vi "Load Instrument Classes.vi"(8 "error in (no error)":errorcluster, 11 "C.E.":refnum<class "Control Experiment.lvclass">) -> (0 "error out":errorcluster, 1 "unresolved":string[](array[string]), 2 "cancelled":bool, 3 "Control Experiment":refnum<class "Control Experiment.lvclass">)   [LabVIEW 2019, in "Control Experiment.lvclass"]
uses:
  Control Experiment.lvclass
  Typedefs/Instrument Class Rings--Cluster.ctl
  <userlib>/LevyLab/Instrument Framework/Instrument/Instrument.lvclass
  C:/Program Files/National Instruments/LabVIEW 2019/vi.lib/JKI/JKI SMO/SMO/SMO.lvclass
  Control Experiment.lvclass/Control Experiment.ctl
  Typedefs/Instrument Classes--cluster.ctl
  <userlib>/LevyLab/Instrument Framework/Instrument Types/Lockin/Instrument.LockinAPI.lvclass
  <userlib>/LevyLab/Instrument Framework/Instrument Types/Amplifier/Instrument.Amplifier.lvclass
  <userlib>/LevyLab/Instrument Framework/Instrument Types/Cryostat/Instrument.Cryostat.lvclass
  <userlib>/LevyLab/Instrument Framework/Instrument Types/CBridge/Instrument.CBridge.lvclass
  <userlib>/LevyLab/Instrument Framework/Instrument Types/Delay Line/Instrument.DelayLine.lvclass
  <userlib>/LevyLab/Instrument Framework/Instrument Types/Strain/Instrument.Strain.lvclass
  <userlib>/LevyLab/Instrument Framework/Instrument Types/VNA/Instrument.VNA.lvclass
  <userlib>/LevyLab/Instrument Framework/Instrument Types/VSource/Instrument.VSource.lvclass
  Typedefs/Instrument Types--enum.ctl
  <userlib>/LevyLab/Instrument Framework/Instrument/Instrument.lvclass/Instrument.ctl
  <vilib>/Utility/Data Type/NI_Data Type.lvlib
  Attributes/Instrument Attributes.lvlib
  <vilib>/JKI/JKI SMO/URI Parsing/URI.lvlib
panel:
  in  "DAQ":refnum<visa-resource-name>
  in  "Instrument Addresses":T1 caption="Instruments"
  in  "OK":bool
  in  "Instrument Classes":T2 {"Amplifier" items=["", "Krohn-Hite-7008"]; "DAQ" items=["", "Lockin"]; "Strain Cell" items=["", "RP100"]; "Capacitance" items=["", "AH2500"]; "Level" items=["", "Cryostation", "OxfordVRM", "OptiCool", "PPMS", "PPMS1", "PPMS2", "PPMS3"]; "Rotator" items=["", "Cryostation", "OxfordVRM", "OptiCool", "PPMS", "PPMS1", "PPMS2", "PPMS3"]; "Magnet" items=["", "Cryostation", "OxfordVRM", "OptiCool", "PPMS", "PPMS1", "PPMS2", "PPMS3"]; "Temperature" items=["", "Cryostation", "OxfordVRM", "OptiCool", "PPMS", "PPMS1", "PPMS2", "PPMS3"]}
  out "Status":string
  # "1. Choose / Confirm Instrument Classes"
  # "2. Choose / Confirm Remote Instruments"
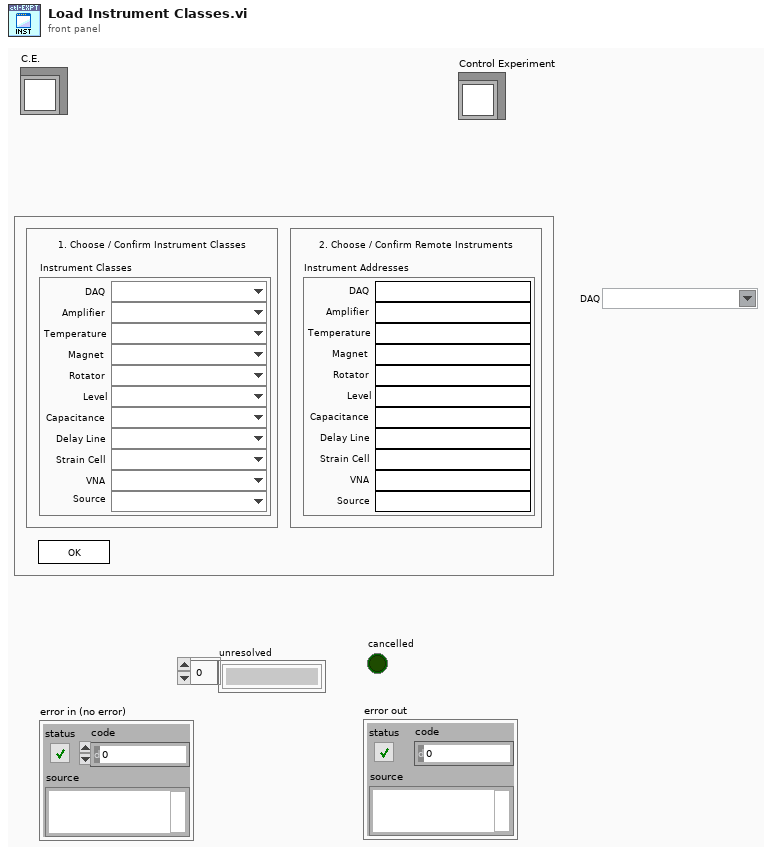
[diagram p1: front panel]
types:
  T1 = cluster{"DAQ":string, "Amplifier":string, "Temperature":string, "Magnet":string, "Rotator":string, "Level":string, "Capacitance Bridge":string, "Delay Line":string, "Strain Cell":string, "VNA":string, "Source":string}
  T2 = typedef "Control Experiment.lvclass/Instrument Class Rings--Cluster.ctl" = cluster{"DAQ":u16, "Amplifier":u16, "Temperature":u16, "Magnet":u16, "Rotator":u16, "Level":u16, "Capacitance":u16, "Delay Line":u16, "Strain Cell":u16, "VNA":u16, "Source":u16}
  T3 = enum32{"Invalid", "Standard", "Closed", "Hidden", "Minimized", "Maximized"}
  T4 = enum32{"invalid app kind", "Development System", "Run Time System", "Student Edition", "Embedded LabVIEW", "Evaluation", "Custom"}
  T5 = typedef "Control Experiment.lvclass/Instrument Classes--cluster.ctl" = cluster{"DAQ":refnum<class "Instrument.LockinAPI.lvclass">, "Amplifier":refnum<class "Instrument.Amplifier.lvclass">, "Temperature":refnum<class "Instrument.Cryostat.lvclass">, "Magnet":refnum<class "Instrument.Cryostat.lvclass">, "Rotator":refnum<class "Instrument.Cryostat.lvclass">, "Level":refnum<class "Instrument.Cryostat.lvclass">, "Capacitance":refnum<class "Instrument.CBridge.lvclass">, "Delay Line":refnum<class "Instrument.DelayLine.lvclass">, "Strain Cell":refnum<class "Instrument.Strain.lvclass">, "VNA":refnum<class "Instrument.VNA.lvclass">, "Source":refnum<class "Instrument.VSource.lvclass">}
  T6 = typedef "Control Experiment.lvclass/Instrument Types--enum.ctl" = enum16{"DAQ", "Amplifier", "Temperature", "Magnet", "Rotator", "Level", "Capacitance", "Delay Line", "Strain Cell", "VNA", "Source"}
  T7 = cluster{"Core":cluster{"Current VI Reference":refnum<vi>, "Close Panel on Exit?":bool}, "C.E.":refnum<class "Control Experiment.lvclass">, "Instruments":refnum<vi>, "Addresses":refnum<vi>, "Instrument Class Rings":refnum<vi>[], "Installed Instruments":refnum<class "Instrument.lvclass">[], "Cast Instruments":refnum<class "Instrument.lvclass">[]}
  T8 = cluster{"Current VI Reference":refnum<vi>, "Close Panel on Exit?":bool}
  T9 = enum32{"Bad", "Idle", "Run top level", "Running"}
  T10 = typedef "Control Experiment.lvclass/Instruments--cluster.ctl" = cluster{"class path":path, "Address":string, "Type":T6}
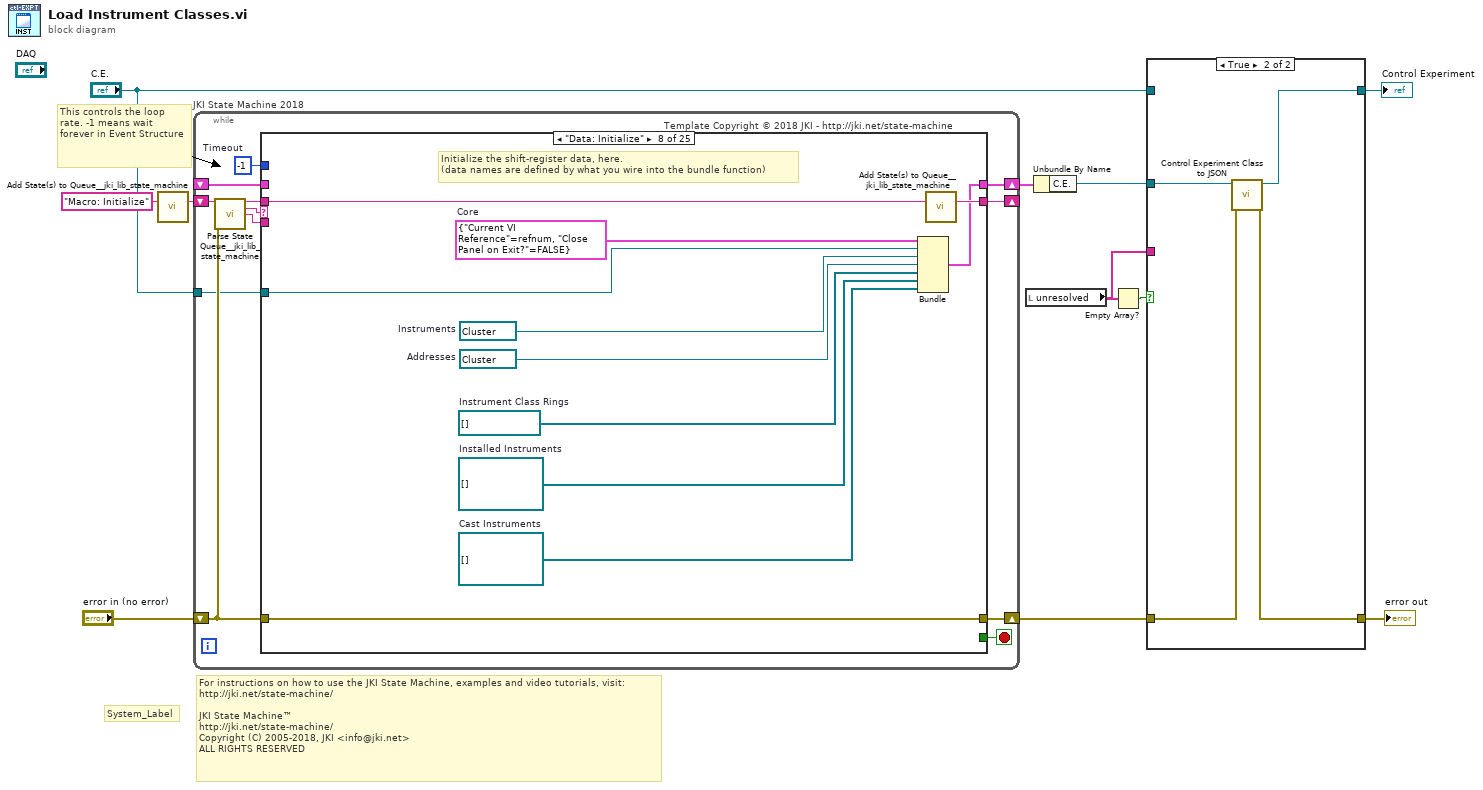
[diagram p0: block diagram]
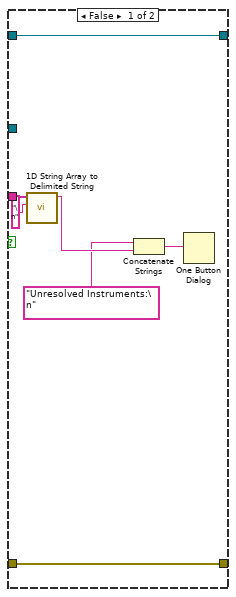
[diagram p2: hidden frame]
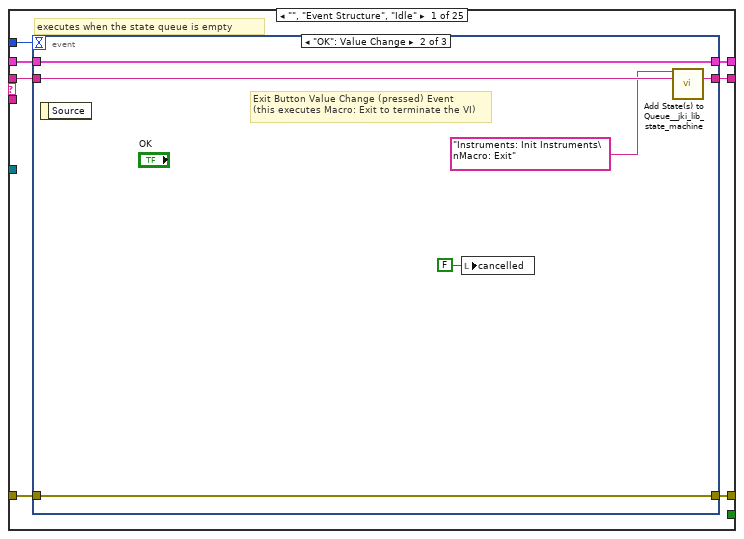
[diagram p3: hidden frame]
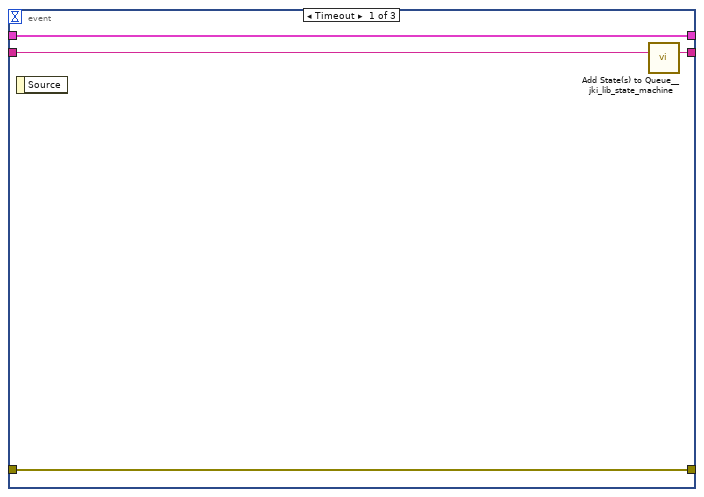
[diagram p4: hidden frame]
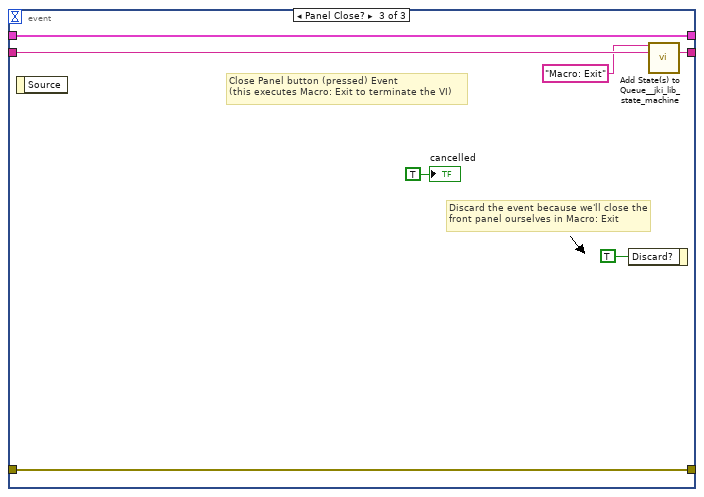
[diagram p5: hidden frame]
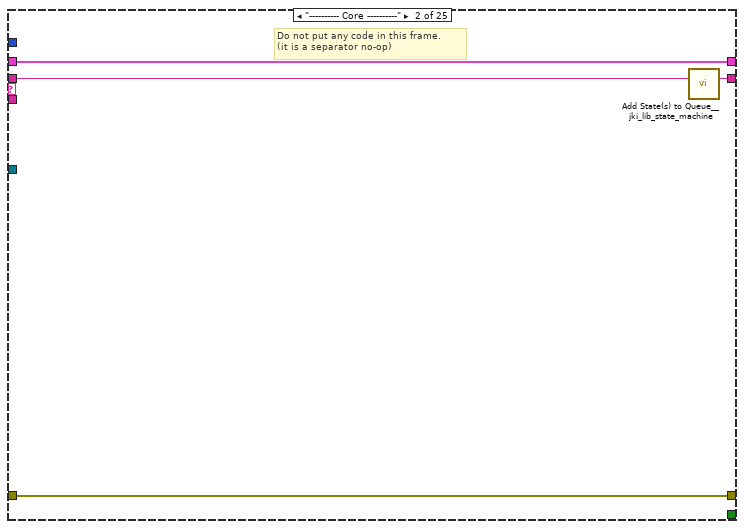
[diagram p6: hidden frame]
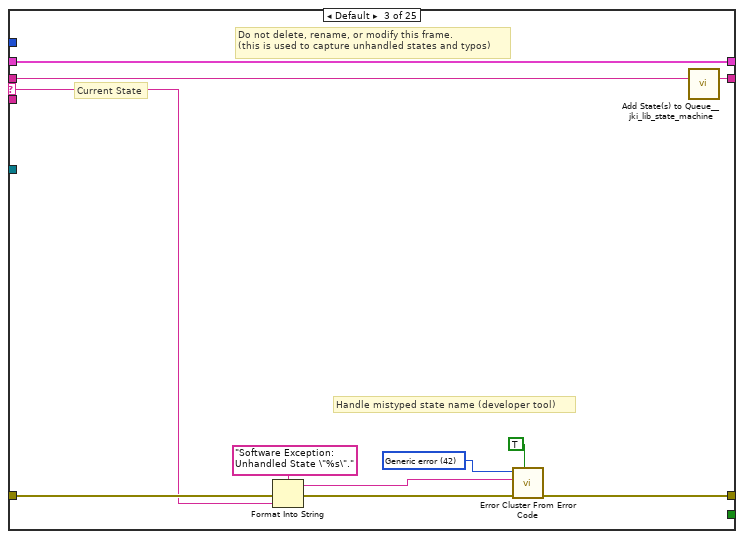
[diagram p7: hidden frame]
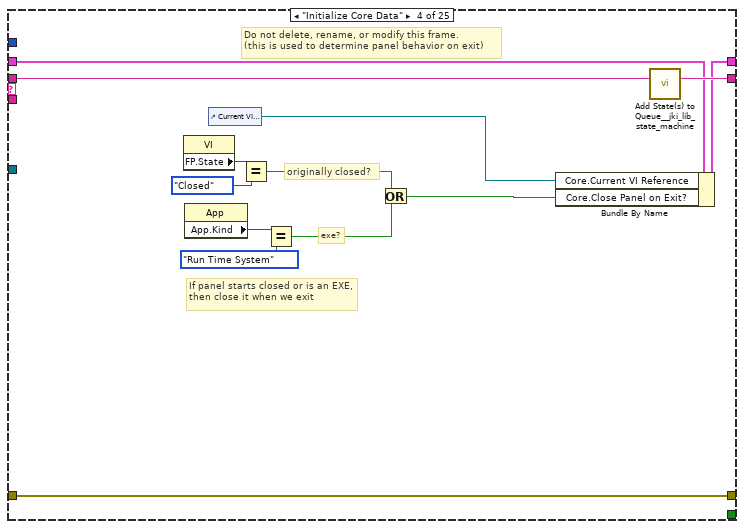
[diagram p8: hidden frame]
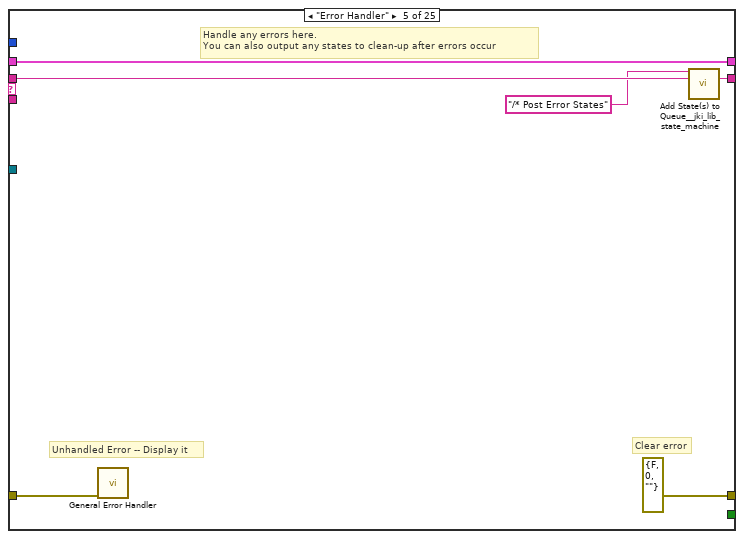
[diagram p9: hidden frame]
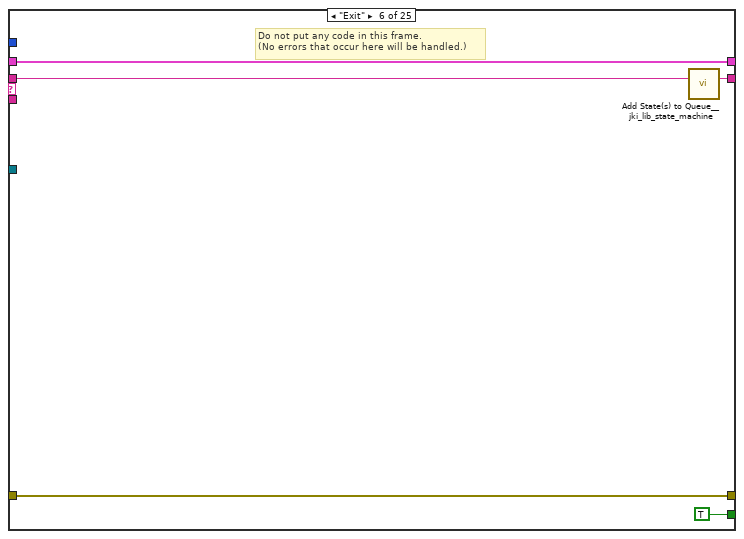
[diagram p10: hidden frame]
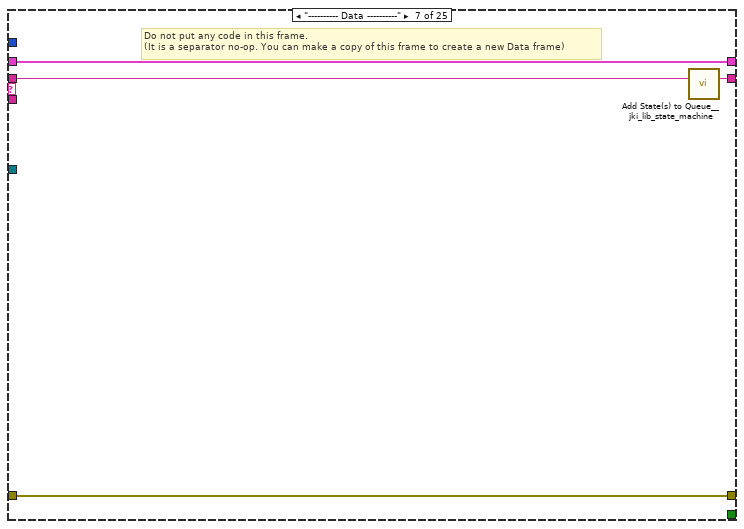
[diagram p11: hidden frame]
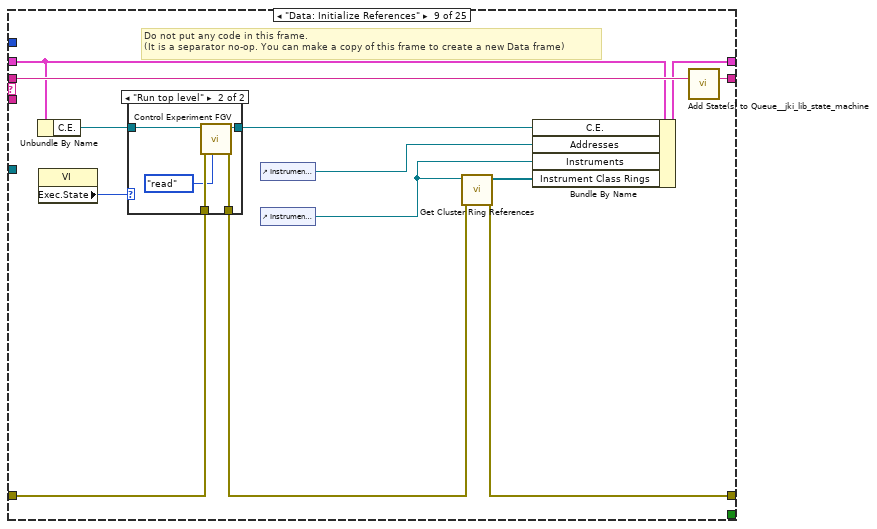
[diagram p12: hidden frame]
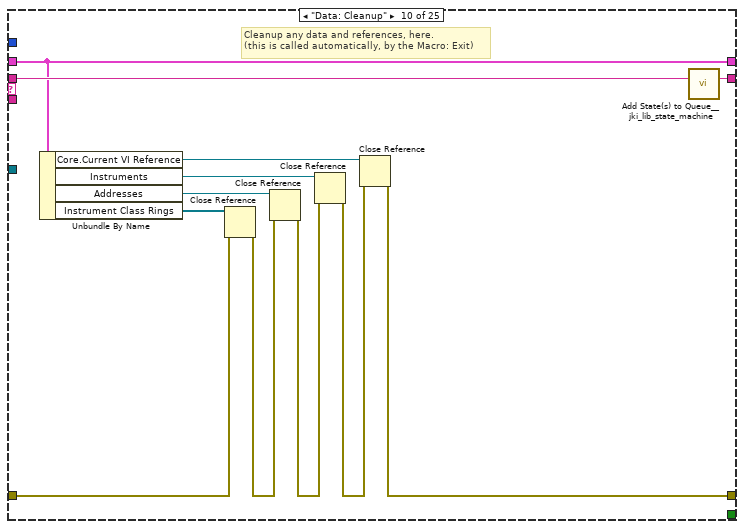
[diagram p14: hidden frame]
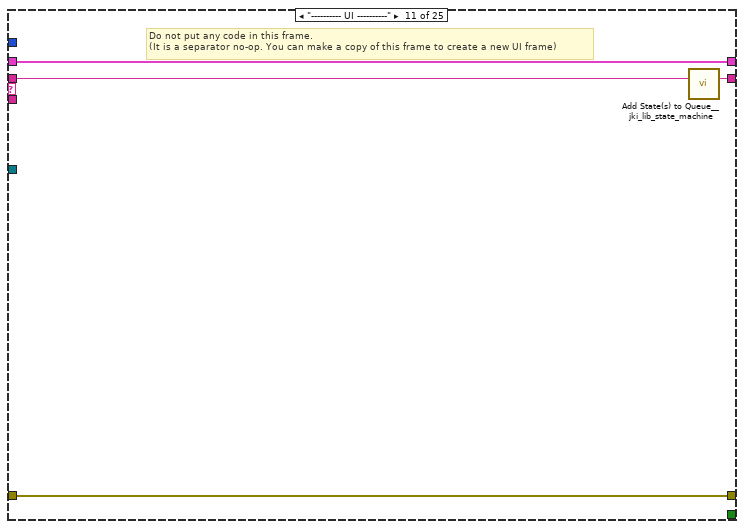
[diagram p15: hidden frame]
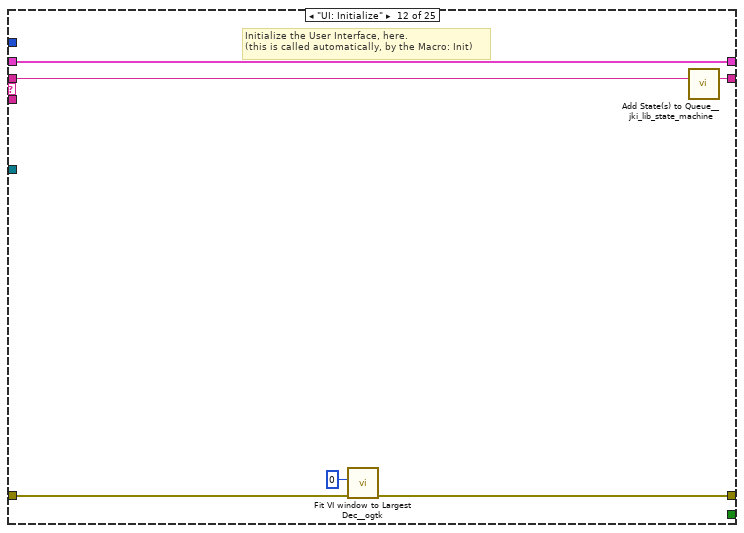
[diagram p16: hidden frame]
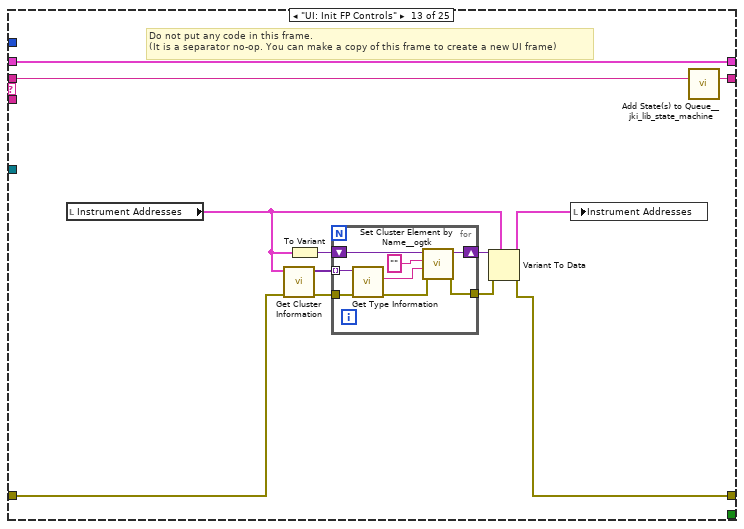
[diagram p17: hidden frame]
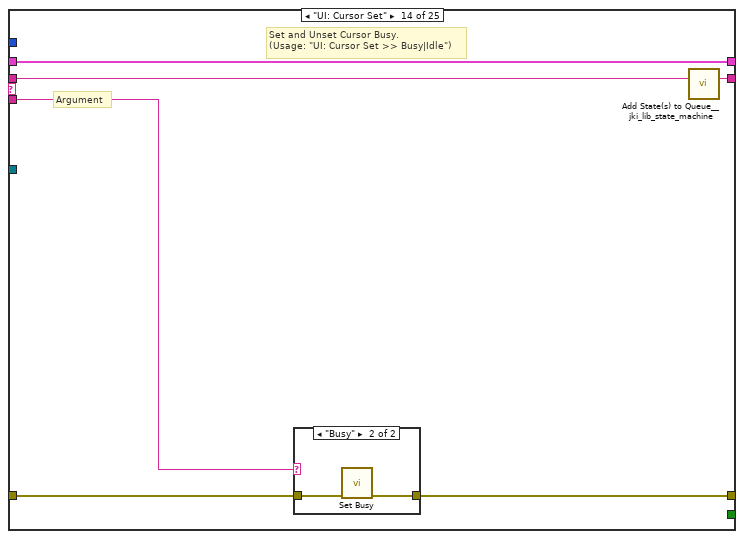
[diagram p18: hidden frame]
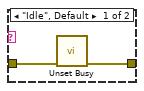
[diagram p19: hidden frame]
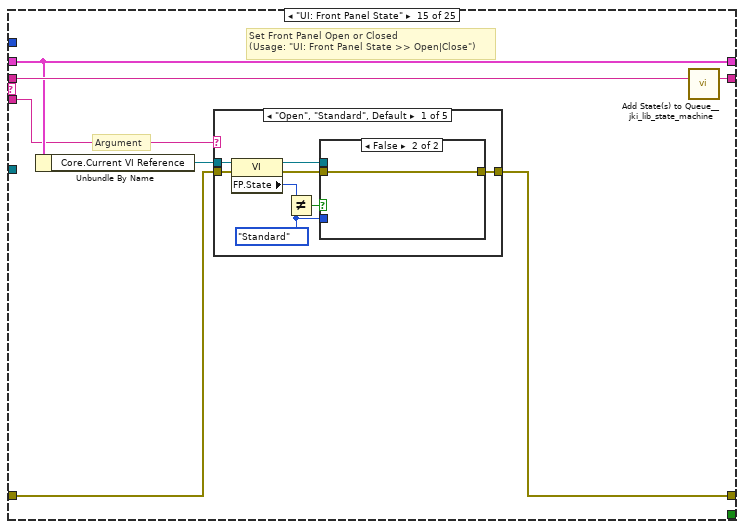
[diagram p20: hidden frame]
diagram:
  # "For instructions on how to use the JKI State Machine, examples and video tutorials, visit:\nhttp://jki.net/state-machine/\n\nJKI State Machine™\nhttp://jki.net/state-machine/\nCopyright (C) 2005-2018, JKI <info@jki.net>\nALL RIGHTS RESERVED"
  # "This controls the loop rate. -1 means wait forever in Event Structure"
  # "System_Label"
  n1 = call <vilib>:"Add State(s) to Queue__jki_lib_state_machine.vi"("State(s) in (\"\")"="Macro: Initialize") -> ("States Out"=w11:string)  [unwired: 14 in]
  n2 = while "JKI State Machine 2018" {
    shift-right: [w16] -> w9
    shift-left: _ -> [w15]
    shift-right: [w19] -> w5
    shift-left: "error in (no error)" -> [w13]
    shift-right: [w18] -> _
    shift-left: w11 -> [w20]
    tunnel: "C.E." -> [w12]
    stop <- w17 stop-if-true
    w14 = -1  # Timeout
    # "Template Copyright © 2018 JKI - http://jki.net/state-machine"
    n3 = call <vilib>:"Parse State Queue__jki_lib_state_machine.vi"("State Queue"=w20, "Error In (no error)"=w13) -> ("Remaining States"=w22:string, "Current State"=w23:string, "Arguments"=w21:string)  [unwired: 11 in]
    n4 = case shown="\"Data: Initialize\"" w23 {
      selector: w23 -> [_ _ w52 _ _ _ _ _ _ _ _ _ _ _ _ _ _ _ _ _ _ _ _ _ _]
      tunnel: w22 -> [w30 w51 w56 w75 w81 w86 w90 w101 w114 w133 w137 w143 w155 w169 w180 w249 w254 w265 w269 w275 w288 w309 w315 w332 w349]
      tunnel: w21 -> [_ _ _ _ _ _ _ _ _ _ _ _ _ w164 w174 _ _ _ _ _ _ _ _ _ _]
      tunnel: w15 -> [w28 w48 w54 w68 w78 w84 w87 _ w107 w129 w134 w139 w149 w167 w176 w246 w251 w262 w266 w272 w281 w302 w312 w329 w343]
      tunnel: [w27 w49 w58 w72 errorcluster {"status"=FALSE, "code"=0, "source"=""} ("error out") w83 w88 w98 w110 w130 w135 w141 w146 w165 w177 w247 w252 w263 w267 w271 w280 w307 w313 w330 w345] -> w19
      tunnel: w13 -> [w26 w49 w57 w72 w77 w83 w88 w98 w108 w125 w135 w140 w145 w166 w178 w247 w252 w263 w267 w270 w280 w306 w313 w330 w335]
      tunnel: [w29 w50 w55 w74 w80 w85 w89 w100 w113 w132 w136 w142 w154 w168 w179 w248 w253 w264 w268 w274 w287 w308 w314 w331 w348] -> w18
      tunnel: [_ _ _ _ _ TRUE _ _ _ _ _ _ _ _ _ _ _ _ _ _ _ _ _ _ _] -> w17
      tunnel: [w25 w48 w54 w73 w78 w84 w87 w99 w112 w129 w134 w139 w149 w167 w176 w246 w251 w262 w266 w272 w282 w302 w312 w329 w344] -> w16
      tunnel: w14 -> [w24 _ _ _ _ _ _ _ _ _ _ _ _ _ _ _ _ _ _ _ _ _ _ _ _]
      tunnel: w12 -> [_ _ _ _ _ _ _ w91 _ _ _ _ _ _ _ _ _ _ _ _ _ _ _ _ _]
      frame "", "Event Structure", "Idle" {
        # "executes when the state queue is empty"
        n5 = event shown="[1] \"OK\": Value Change" {
          selector: _ -> [_ _ _]
          dyn-events: _ -> [_ _ _]
          timeout: w24 -> [_ _ _]
          tunnel: w30 -> [w34 w40 w47]
          tunnel: [w33 w39 w46] -> w29
          tunnel: w28 -> [w31 w37 w44]
          tunnel: [w32 w38 w45] -> w27
          tunnel: w26 -> [w32 w38 w45]
          tunnel: [w31 w37 w44] -> w25
          event Timeout {
            n6 = event-data() -> ()  [unwired: 1 in, 1 out]
            n7 = call <vilib>:"Add State(s) to Queue__jki_lib_state_machine.vi"("State(s) in (\"\")"=w34) -> ("States Out"=w33:string)  [unwired: 14 in]
          }
          event "OK": Value Change {
            # "Exit Button Value Change (pressed) Event\n(this executes Macro: Exit to terminate the VI)"
            n8 = event-data() -> ()  [unwired: 1 in, 1 out]
            n9 = local write "cancelled"(FALSE ("cancelled")) -> ()
            n10 = call <vilib>:"Add State(s) to Queue__jki_lib_state_machine.vi"("State(s) in Front (\"\")"="Instruments: Init Instruments\nMacro: Exit", "State(s) in (\"\")"=w40) -> ("States Out"=w39:string)  [unwired: 13 in]
          }
          event Panel Close? {
            # "Discard the event because we'll close the front panel ourselves in Macro: Exit"
            # "Close Panel button (pressed) Event\n(this executes Macro: Exit to terminate the VI)"
            n11 = event-data() -> ()  [unwired: 1 in, 1 out]
            n12 = event-data("Discard?"=TRUE) -> ()  [unwired: 1 in, 1 out]
            n13 = call <vilib>:"Add State(s) to Queue__jki_lib_state_machine.vi"("State(s) in Front (\"\")"="Macro: Exit", "State(s) in (\"\")"=w47) -> ("States Out"=w46:string)  [unwired: 13 in]
            "cancelled" <- TRUE ("cancelled")
          }
        }
      }
      frame "---------- Core ----------" {
        # "Do not put any code in this frame.\n(it is a separator no-op)"
        n14 = call <vilib>:"Add State(s) to Queue__jki_lib_state_machine.vi"("State(s) in (\"\")"=w51) -> ("States Out"=w50:string)  [unwired: 14 in]
      }
      frame Default {
        w61 = 42 items=["No error", "Argument error", "Memory is full", "Out of zone", "End of file", "File already open", "Generic file I/O error", "File not found", "File permission error", "Disk is full", "Duplicate path", "Too many files open", "System feature not enabled", "Resource file not found", "Cannot add resource", "Resource not found", "Image not found", "Image memory error", "Pen does not exist", "Config type invalid", "Config token not found", "Config parse error", "Config memory error", "Bad external code format", "Bad external code offset", "External code not present", "Null window", "Destroy window error", "Null menu", "Print aborted", "Bad print record", "Print driver error", "Windows error during printing", "Memory error during printing", "Print dialog error", "Generic print error", "Invalid device refnum", "Device not found", "Device parameter error", "Device unit error", "Cannot open device", "Device call aborted", "Generic error", "Cancelled by user", "Object ID too low", "Object ID too high", "Object not in heap", "Unknown heap", "Unknown object (invalid DefProc)", "Unknown object (DefProc not in table)", "Message out of range", "Invalid (null) method", "Unknown message", "Manager call not supported", "Bad address", "Network operation in progress", "Network operation timed out", "Connection is busy", "Network attribute not supported", "Network error", "Address in use", "System out of memory", "Connection aborted", "Connection refused", "Not connected", "Already connected", "Connection closed", "Initialization error (interapplication manager)", "Bad occurrence", "Wait on unbound occurrence handler", "Occurrence queue overflow", "Datalog type conflict", "Unused", "Unrecognized type (interapplication manager)", "Memory corrupt", "Failed to make temporary DLL", "Old CIN version", "Drag socket not found", "Failed to load drop-object", "Failed to register OLE object", "Failed to release OLE object", "Format specifier type mismatch", "Unknown format specifier", "Too few format specifiers", "Too many format specifiers", "Scan failed", "Newer CIN version", "Error converting to variant", "Runtime menu error", "Password tampered", "Variant attribute not found", "Incompatible variant data type", "Event data is not available", "Event Store is not present", "Occurrence is not found", "Event Queue is not created", "Event info is not available", "Refnum passed is NULL", "Error retrieving Class GUID", "Error retrieving CoClass GUID", "Error retrieving TypeLib GUID.", "Bad built application magic bytes.", "Specific driver is different from the specific driver associated with the Logical Name.", "There is no session opened to the class driver.", "Max Error", "MAX - Error with config objects", "MAX - Error loading configuration", "MAX - Group not supported"]
        # "Current State"
        # "Do not delete, rename, or modify this frame.\n(this is used to capture unhandled states and typos)"
        # "Handle mistyped state name (developer tool)"
        n15 = Format Into String(format string="Software Exception: Unhandled State \"%s\"." ("message"), error in=w57, w52) -> (resulting string=w60:string, error out=w59:errorcluster)  [unwired: 1 in]
        n16 = call <vilib>:"Error Cluster From Error Code.vi"("show call chain? (False)"=TRUE, "error in (no error)"=w59, "error message (\"\")"=w60, "error code (0)"=w61) -> ("error out"=w58:errorcluster)  [unwired: 5 in]
        n17 = call <vilib>:"Add State(s) to Queue__jki_lib_state_machine.vi"("State(s) in (\"\")"=w56) -> ("States Out"=w55:string)  [unwired: 14 in]
      }
      frame "Initialize Core Data" {
        # "Do not delete, rename, or modify this frame.\n(this is used to determine panel behavior on exit)"
        # "originally closed?"
        # "exe?"
        # "If panel starts closed or is an EXE, then close it when we exit"
        n18 = property class="VI"() -> ("FP.State"=w65:T3)  [unwired: 2 in, 2 out]
        n19 = property class="App"() -> ("App.Kind"=w71:T4)  [unwired: 2 in, 2 out]
        n20 = control-ref of="Current VI Reference"() -> (w66:refnum<vi>)
        n21 = Equal?(x=w65, y=T3."Closed" ("Front Panel Window:State")) -> (x = y?=w63:bool)
        n22 = Equal?(x=w71, y=T4."Run Time System" ("Application:Kind")) -> (x = y?=w69:bool)
        n23 = Or(x=w63, y=w69) -> (x .or. y?=w67:bool)
        n24 = Bundle By Name(cluster=w68, "Core.Current VI Reference"=w66, "Core.Close Panel on Exit?"=w67) -> (w73:T7)
        n25 = call <vilib>:"Add State(s) to Queue__jki_lib_state_machine.vi"("State(s) in (\"\")"=w75) -> ("States Out"=w74:string)  [unwired: 14 in]
      }
      frame "Error Handler" {
        # "Unhandled Error -- Display it"
        # "Handle any errors here.\nYou can also output any states to clean-up after errors occur"
        # "Clear error"
        n26 = call <vilib>:"General Error Handler.vi"("error in (no error)"=w77) -> ()  [unwired: 10 in, 5 out]
        n27 = call <vilib>:"Add State(s) to Queue__jki_lib_state_machine.vi"("State(s) in Front (\"\")"="/* Post Error States", "State(s) in (\"\")"=w81) -> ("States Out"=w80:string)  [unwired: 13 in]
      }
      frame "Exit" {
        # "Do not put any code in this frame.\n(No errors that occur here will be handled.)"
        n28 = call <vilib>:"Add State(s) to Queue__jki_lib_state_machine.vi"("State(s) in (\"\")"=w86) -> ("States Out"=w85:string)  [unwired: 14 in]
      }
      frame "---------- Data ----------" {
        # "Do not put any code in this frame.\n(It is a separator no-op. You can make a copy of this frame to create a new Data frame)"
        n29 = call <vilib>:"Add State(s) to Queue__jki_lib_state_machine.vi"("State(s) in (\"\")"=w90) -> ("States Out"=w89:string)  [unwired: 14 in]
      }
      frame "Data: Initialize" {
        w92 = refnum<vi> refnum  # Addresses
        w93 = refnum<vi> refnum  # Instruments
        w94 = refnum<class "Instrument.lvclass">[] []  # Cast Instruments
        w95 = refnum<vi>[] []  # Instrument Class Rings
        w96 = refnum<class "Instrument.lvclass">[] []  # Installed Instruments
        w97 = T8 {"Current VI Reference"=refnum, "Close Panel on Exit?"=FALSE}  # Core
        # "Initialize the shift-register data, here.\n(data names are defined by what you wire into the bundle function)"
        n30 = Bundle("Core"=w97, "C.E."=w91, "Instruments"=w93, "Addresses"=w92, "Instrument Class Rings"=w95, "Installed Instruments"=w96, "Cast Instruments"=w94) -> (w99:T7)  [unwired: 1 in]
        n31 = call <vilib>:"Add State(s) to Queue__jki_lib_state_machine.vi"("State(s) in (\"\")"=w101) -> ("States Out"=w100:string)  [unwired: 14 in]
      }
      frame "Data: Initialize References" {
        # "Do not put any code in this frame.\n(It is a separator no-op. You can make a copy of this frame to create a new Data frame)"
        n32 = Unbundle By Name(w107) -> ("C.E."=w106:refnum<class "Control Experiment.lvclass">)
        n33 = property class="VI"() -> ("Exec.State"=w105:T9)  [unwired: 2 in, 2 out]
        n34 = case shown="\"Run top level\"" w105 {
          tunnel: [w115 w121] -> w109
          tunnel: w108 -> [w115 w120]
          tunnel: [w116 w118] -> w103
          tunnel: w106 -> [w116 w117]
          frame Default {
          }
          frame "Run top level" {
            n35 = call "Control Experiment FGV.vi"("Function"=enum16{"read", "write"}."read", "error in (no error)"=w120, "Control Experiment.lvclass"=w117) -> ("error out"=w121:errorcluster, "Control Experiment.lvclass out"=w118:refnum<class "Control Experiment.lvclass">)  [unwired: 5 in, 2 out]
          }
        }
        n36 = control-ref of="Instrument Addresses"() -> (w104:refnum<vi>)
        n37 = control-ref of="Instrument Classes"() -> (w102:refnum<vi>)
        n38 = call "Get Cluster Ring References.vi"("error in (no error)"=w109, "Cluster Reference in"=w102) -> ("error out"=w110:errorcluster, "Ring References"=w111:refnum<vi>[])  [unwired: 8 in]
        n39 = Bundle By Name(cluster=w107, "C.E."=w103, "Addresses"=w104, "Instruments"=w102, "Instrument Class Rings"=w111) -> (w112:T7)
        n40 = call <vilib>:"Add State(s) to Queue__jki_lib_state_machine.vi"("State(s) in (\"\")"=w114) -> ("States Out"=w113:string)  [unwired: 14 in]
      }
      frame "Data: Cleanup" {
        # "Cleanup any data and references, here.\n(this is called automatically, by the Macro: Exit)"
        n41 = Unbundle By Name(w129) -> ("Core.Current VI Reference"=w131:refnum<vi>, "Instruments"=w128:refnum<vi>, "Addresses"=w127:refnum<vi>, "Instrument Class Rings"=w126:refnum<vi>[])
        n42 = Close Reference(reference=w126, error in (no error)=w125) -> (error out=w124:errorcluster)
        n43 = Close Reference(reference=w127, error in (no error)=w124) -> (error out=w123:errorcluster)
        n44 = Close Reference(reference=w128, error in (no error)=w123) -> (error out=w122:errorcluster)
        n45 = Close Reference(reference=w131, error in (no error)=w122) -> (error out=w130:errorcluster)
        n46 = call <vilib>:"Add State(s) to Queue__jki_lib_state_machine.vi"("State(s) in (\"\")"=w133) -> ("States Out"=w132:string)  [unwired: 14 in]
      }
      frame "---------- UI ----------" {
        # "Do not put any code in this frame.\n(It is a separator no-op. You can make a copy of this frame to create a new UI frame)"
        n47 = call <vilib>:"Add State(s) to Queue__jki_lib_state_machine.vi"("State(s) in (\"\")"=w137) -> ("States Out"=w136:string)  [unwired: 14 in]
      }
      frame "UI: Initialize" {
        # "Initialize the User Interface, here.\n(this is called automatically, by the Macro: Init)"
        n48 = call <userlib>:"Fit VI window to Largest Dec__ogtk.vi"("error in (no error)"=w140, "border spacing (2 px)"=0) -> ("error out"=w141:errorcluster)  [unwired: 4 in, 1 out]
        n49 = call <vilib>:"Add State(s) to Queue__jki_lib_state_machine.vi"("State(s) in (\"\")"=w143) -> ("States Out"=w142:string)  [unwired: 14 in]
      }
      frame "UI: Init FP Controls" {
        # "Do not put any code in this frame.\n(It is a separator no-op. You can make a copy of this frame to create a new UI frame)"
        n50 = local read "Instrument Addresses"() -> (w144:T1)
        n51 = call <vilib>:"Get Cluster Information.vi"("error in (no error)"=w145, "variant"=w144) -> ("error out"=w151:errorcluster, "cluster elements"=w153:variant[])  [unwired: 8 in]
        n52 = To Variant(anything=w144) -> (Variant=w148:variant)
        n53 = for {
          tunnel: w153 -> [w163] mode=indexing
          shift-right: [w161] -> w152
          shift-left: w148 -> [w162]
          tunnel: w151 -> [w156]
          tunnel: [w157] -> w150
          n54 = call <vilib>:"Get Type Information.vi"("error in (no error)"=w156, "variant"=w163) -> ("error out"=w158:errorcluster, "name"=w159:string)  [unwired: 5 in, 3 out]
          n55 = call <userlib>:"Set Cluster Element by Name__ogtk.vi"("error in (no error)"=w158, "Element Name (\"\": New Element Data Name)"=w159, "New Element Value"="", "Cluster"=w162) -> ("error out"=w157:errorcluster, "VCluster out"=w161:variant)  [unwired: 5 in, 1 out]
        }
        n56 = Variant To Data(error in=w150, type=w144, Variant=w152) -> (data=w147:T1, error out=w146:errorcluster)
        n57 = local write "Instrument Addresses"(w147) -> ()
        n58 = call <vilib>:"Add State(s) to Queue__jki_lib_state_machine.vi"("State(s) in (\"\")"=w155) -> ("States Out"=w154:string)  [unwired: 14 in]
      }
      frame "UI: Cursor Set" {
        # "Argument"
        # "Set and Unset Cursor Busy.\n(Usage: \"UI: Cursor Set >> Busy|Idle\")"
        n59 = case shown="\"Busy\"" w164 {
          tunnel: w166 -> [w171 w173]
          tunnel: [w170 w172] -> w165
          frame "Idle", Default {
            n60 = call <vilib>:"Unset Busy.vi"("error in (no error)"=w171) -> ("error out"=w170:errorcluster)  [unwired: 10 in]
          }
          frame "Busy" {
            n61 = call <vilib>:"Set Busy.vi"("error in (no error)"=w173) -> ("error out"=w172:errorcluster)  [unwired: 9 in, 1 out]
          }
        }
        n62 = call <vilib>:"Add State(s) to Queue__jki_lib_state_machine.vi"("State(s) in (\"\")"=w169) -> ("States Out"=w168:string)  [unwired: 14 in]
      }
      frame "UI: Front Panel State" {
        # "Argument"
        # "Set Front Panel Open or Closed\n(Usage: \"UI: Front Panel State >> Open|Close\")"
        n63 = Unbundle By Name(w176) -> ("Core.Current VI Reference"=w175:refnum<vi>)
        n64 = case shown="\"Open\", \"Standard\", Default" w174 {
          tunnel: w178 -> [w186 w201 w212 w225 w238]
          tunnel: [w188 w202 w214 w227 w240] -> w177
          tunnel: w175 -> [w187 w199 w213 w226 w239]
          frame "Open", "Standard", Default {
            w181 = T3."Standard" ("State")
            n65 = property class="VI"(reference=w187, error in=w186) -> (reference out=w184:refnum<vi>, error out=w185:errorcluster, "FP.State"=w183:T3)
            n66 = Not Equal?(x=w183, y=w181) -> (x != y?=w182:bool)
            n67 = case shown="False" w182 {
              tunnel: [w192 w194] -> w188
              tunnel: w185 -> [w191 w194]
              tunnel: w184 -> [w190 _]
              tunnel: w181 -> [w189 _]
              frame True {
                n68 = invoke class="VI" method="FP.Open"(reference=w190, error in=w191, "Activate"=TRUE, "State"=w189) -> (error out=w192:errorcluster)  [unwired: 1 in, 4 out]
              }
              frame False {
              }
            }
          }
          frame "Close", "Closed" {
            n69 = property class="VI"(reference=w199, error in=w201) -> (reference out=w198:refnum<vi>, error out=w200:errorcluster, "FP.State"=w196:T3)
            n70 = Not Equal?(x=w196, y=T3."Closed" ("Front Panel Window:State")) -> (x != y?=w195:bool)
            n71 = case shown="True" w195 {
              tunnel: [w203 w206] -> w202
              tunnel: w200 -> [w203 w205]
              tunnel: w198 -> [_ w204]
              frame False {
              }
              frame True {
                n72 = invoke class="VI" method="FP.Close"(reference=w204, error in=w205) -> (error out=w206:errorcluster)  [unwired: 1 in, 2 out]
              }
            }
          }
          frame "Hidden", "Hide" {
            w207 = T3."Hidden" ("State")
            n73 = property class="VI"(reference=w213, error in=w212) -> (reference out=w210:refnum<vi>, error out=w211:errorcluster, "FP.State"=w209:T3)
            n74 = Not Equal?(x=w209, y=w207) -> (x != y?=w208:bool)
            n75 = case shown="True" w208 {
              tunnel: [w218 w219] -> w214
              tunnel: w211 -> [w217 w219]
              tunnel: w210 -> [w216 _]
              tunnel: w207 -> [w215 _]
              frame True {
                n76 = invoke class="VI" method="FP.Open"(reference=w216, error in=w217, "State"=w215) -> (error out=w218:errorcluster)  [unwired: 2 in, 4 out]
              }
              frame False {
              }
            }
          }
          frame "Minimize", "Minimized" {
            w220 = T3."Minimized" ("State")
            n77 = property class="VI"(reference=w226, error in=w225) -> (reference out=w223:refnum<vi>, error out=w224:errorcluster, "FP.State"=w222:T3)
            n78 = Not Equal?(x=w222, y=w220) -> (x != y?=w221:bool)
            n79 = case shown="True" w221 {
              tunnel: [w231 w232] -> w227
              tunnel: w224 -> [w230 w232]
              tunnel: w223 -> [w229 _]
              tunnel: w220 -> [w228 _]
              frame True {
                n80 = invoke class="VI" method="FP.Open"(reference=w229, error in=w230, "State"=w228) -> (error out=w231:errorcluster)  [unwired: 2 in, 4 out]
              }
              frame False {
              }
            }
          }
          frame "Maximize", "Maximized" {
            w233 = T3."Maximized" ("State")
            n81 = property class="VI"(reference=w239, error in=w238) -> (reference out=w236:refnum<vi>, error out=w237:errorcluster, "FP.State"=w235:T3)
            n82 = Not Equal?(x=w235, y=w233) -> (x != y?=w234:bool)
            n83 = case shown="True" w234 {
              tunnel: [w244 w245] -> w240
              tunnel: w237 -> [w243 w245]
              tunnel: w236 -> [w242 _]
              tunnel: w233 -> [w241 _]
              frame True {
                n84 = invoke class="VI" method="FP.Open"(reference=w242, error in=w243, "State"=w241) -> (error out=w244:errorcluster)  [unwired: 2 in, 4 out]
              }
              frame False {
              }
            }
          }
        }
        n85 = call <vilib>:"Add State(s) to Queue__jki_lib_state_machine.vi"("State(s) in (\"\")"=w180) -> ("States Out"=w179:string)  [unwired: 14 in]
      }
      frame "---------- Macro ----------" {
        # "Do not put any code in this frame.\n(It is a separator no-op. You can make a copy of this frame to create a new Macro frame)"
        n86 = call <vilib>:"Add State(s) to Queue__jki_lib_state_machine.vi"("State(s) in (\"\")"=w249) -> ("States Out"=w248:string)  [unwired: 14 in]
      }
      frame "Macro: Initialize" {
        # "Initialization Macro\n(This is called once, when the VI starts)"
        n87 = call <vilib>:"Add State(s) to Queue__jki_lib_state_machine.vi"("State(s) in Front (\"\")"="Data: Initialize\nInitialize Core Data\nUI: Initialize\nUI: Front Panel State >> Open\n\nData: Initialize References\nUI: Init FP Controls\n\nRings: Empty Rings\nRings: List Installed\nRings: Installed to Rings\n\nRings: Init Addresses", "State(s) in (\"\")"=w254) -> ("States Out"=w253:string)  [unwired: 13 in]
      }
      frame "Macro: Exit" {
        # "Exit Macro\n(This is called once, when the VI exits)"
        n88 = Unbundle By Name(w262) -> ("Core.Close Panel on Exit?"=w261:bool)
        n89 = Select(t="UI: Front Panel State >> Close", s=w261, f="") -> (s? t:f=w258:string)
        n90 = call <vilib>:"Add State(s) to Queue__jki_lib_state_machine.vi"("State(s) in Front (\"\")"="" ("State(s) in Front (\"\")"), "State(s) in (\"\")"=w258, "State(s) at Back (\"\")"="Data: Cleanup\nExit") -> ("States Out"=w256:string)  [unwired: 12 in]
        n91 = call <vilib>:"Add State(s) to Queue__jki_lib_state_machine.vi"("State(s) in Front (\"\")"=w256, "State(s) in (\"\")"=w265) -> ("States Out"=w264:string)  [unwired: 13 in]
      }
      frame "---------- Rings ----------" {
        # "Template Separator\n(You can make a copy of, or modify, this frame)"
        n92 = call <vilib>:"Add State(s) to Queue__jki_lib_state_machine.vi"("State(s) in (\"\")"=w269) -> ("States Out"=w268:string)  [unwired: 14 in]
      }
      frame "Rings: Empty Rings" {
        # "Template Separator\n(You can make a copy of, or modify, this frame)"
        n93 = Unbundle By Name(w272) -> ("Instrument Class Rings"=w273:refnum<vi>[])
        n94 = call "Empty Rings.vi"("error in (no error)"=w270, "Ring References"=w273) -> ("error out"=w271:errorcluster)  [unwired: 8 in, 1 out]
        n95 = call <vilib>:"Add State(s) to Queue__jki_lib_state_machine.vi"("State(s) in (\"\")"=w275) -> ("States Out"=w274:string)  [unwired: 14 in]
      }
      frame "Rings: List Installed" {
        # "List all classes in \\user.lib\\LevyLab\n(but not \\user.lib\\LevyLab\\Instrument Framework\\\nor Build Support\\)"
        # "Your code here.\n(You can make a copy of, or modify, this frame)"
        n96 = call "Application user.lib.vi"() -> ("path out"=w277:path)  [unwired: 10 in, 1 out]
        n97 = Build Path(base path=w277, name or relative path="LevyLab") -> (appended path=w276:path)
        n98 = call <vilib>:"Recursive File List.vi"("Folders to Exclude"=string[] ["Instrument Framework", "Build Support"], "pattern"="*.lvclass", "Folder Path"=w276) -> ("All Files in Dir"=w286:path[])  [unwired: 4 in, 4 out]
        n99 = for {
          tunnel: w286 -> [w293] mode=indexing
          tunnel: [w298] -> w279 mode=indexing if=w296
          tunnel: w280 -> [w295]
          tunnel: ["" ("String 2")] -> w278
          # "Find children of Instrument"
          n100 = call <vilib>:"Get LV Class Default Value.vi"("error in (no error)"=w295, "class path"=w293) -> ("error out"=w300:errorcluster, "object"=w301:refnum<class>)  [unwired: 8 in]
          n101 = To More Specific Class(target class=refnum<class "Instrument.lvclass"> refnum ("Instrument"), reference=w301, error in=w300) -> (specific class reference=w298:refnum<class "Instrument.lvclass">, error out=w289:errorcluster)
          n102 = Format Into String(format string="Loading...%s", w293) -> (resulting string=→"Status":string)  [unwired: 2 in, 1 out]
          n103 = Unbundle By Name(w289) -> ("status"=w299:bool)
          n104 = Wait (ms)(milliseconds to wait=u32 5) -> ()  [unwired: 1 out]
          n105 = Not(x=w299) -> (.not. x?=w296:bool)
        }
        n106 = Bundle By Name(cluster=w281, "Installed Instruments"=w279) -> (w282:T7)
        n107 = local write "Status"(w278) -> ()
        n108 = call <vilib>:"Add State(s) to Queue__jki_lib_state_machine.vi"("State(s) in (\"\")"=w288) -> ("States Out"=w287:string)  [unwired: 14 in]
      }
      frame "Rings: Installed to Rings" {
        # "Your code here.\n(You can make a copy of, or modify, this frame)"
        n109 = Unbundle By Name(w302) -> ("C.E."=w305:refnum<class "Control Experiment.lvclass">, "Instrument Class Rings"=w303:refnum<vi>[], "Installed Instruments"=w304:refnum<class "Instrument.lvclass">[])
        n110 = call "Installed Classes to Rings.vi"("error in (no error)"=w306, "Installed"=w304, "Rings"=w303, "C.E."=w305) -> ("error out"=w307:errorcluster)  [unwired: 6 in, 1 out]
        n111 = call <vilib>:"Add State(s) to Queue__jki_lib_state_machine.vi"("State(s) in (\"\")"=w309) -> ("States Out"=w308:string)  [unwired: 14 in]
      }
      frame "Rings: Init Addresses" {
        # "Template Separator\n(You can make a copy of, or modify, this frame)"
        n112 = Unbundle By Name(w312) -> ("C.E."=w310:refnum<class "Control Experiment.lvclass">)
        n113 = Unbundle By Name(w310) -> ("Instruments"=w311:T10[])
        n114 = for {
          tunnel: w311 -> [w328] mode=indexing
          n115 = Unbundle By Name(w328) -> ("Address"=w322:string, "Type"=w324:T6)
          n116 = local read "Instrument Addresses"() -> (w323:T1)
          n117 = call <vilib>:"Parse URI.vi"("URI"=w322) -> ("address"=w316:string)  [unwired: 6 in, 4 out]
          n118 = Format Into String(w324) -> (resulting string=w321:string)  [unwired: 3 in, 1 out]
          n119 = Equal?(x="localhost", y=w316) -> (x = y?=w319:bool)
          n120 = Select(t="", s=w319, f=w316) -> (s? t:f=w318:string)
          n121 = call <userlib>:"Set Cluster Element by Name__ogtk.vi"("Element Name (\"\": New Element Data Name)"=w321, "New Element Value"=w318, "Cluster"=w323) -> ("error out"=w327:errorcluster, "VCluster out"=w326:variant)  [unwired: 6 in, 1 out]
          n122 = Variant To Data(error in=w327, type=w323, Variant=w326) -> (data=w325:T1)  [unwired: 1 out]
          n123 = local write "Instrument Addresses"(w325) -> ()
        }
        n124 = call <vilib>:"Add State(s) to Queue__jki_lib_state_machine.vi"("State(s) in (\"\")"=w315) -> ("States Out"=w314:string)  [unwired: 14 in]
      }
      frame "---------- Instruments ----------" {
        # "Template Separator\n(You can make a copy of, or modify, this frame)"
        n125 = call <vilib>:"Add State(s) to Queue__jki_lib_state_machine.vi"("State(s) in (\"\")"=w332) -> ("States Out"=w331:string)  [unwired: 14 in]
      }
      frame "Instruments: Init Instruments" {
        # "#148 clear instrument classes after\nreading previously installed"
        # "Template Separator\n(You can make a copy of, or modify, this frame)"
        n126 = Unbundle By Name(w343) -> ("C.E."=w339:refnum<class "Control Experiment.lvclass">, "Installed Instruments"=w346:refnum<class "Instrument.lvclass">[], "Instrument Class Rings"=w347:refnum<vi>[])
        n127 = Bundle By Name(cluster=w339, "Instrument Classes"=T5 {"DAQ"=refnum, "Amplifier"=refnum, "Temperature"=refnum, "Magnet"=refnum, "Rotator"=refnum, "Level"=refnum, "Capacitance"=refnum, "Delay Line"=refnum, "Strain Cell"=refnum, "VNA"=refnum, "Source"=refnum}) -> (w338:refnum<class "Control Experiment.lvclass">)
        n128 = call <userlib>:"Get Cluster Element Names__ogtk.vi"("error in (no error)"=w335, "Cluster"="Instrument Addresses") -> ("error out"=w334:errorcluster, "Element Names"=w337:string[])  [unwired: 8 in]
        n129 = for {
          tunnel: "Instrument Addresses" -> [w357]
          tunnel: w347 -> [w364] mode=indexing
          shift-right: [w367] -> w341
          shift-left: w338 -> [w368]
          tunnel: w334 -> [w358]
          tunnel: w346 -> [w366]
          tunnel: [w365] -> w342 mode=indexing
          tunnel: w337 -> [w359] mode=indexing
          tunnel: [w351] -> w333 mode=indexing if=w350
          n130 = property class="Ring"(reference=w364) -> ("RingText.Text"=w360:string, "Label.Text"=w363:string)  [unwired: 1 in, 2 out]
          n131 = call <userlib>:"Get Cluster Element by Name__ogtk.vi"("error in (no error)"=w358, "Element Name"=w359, "Cluster"=w357) -> ("error out"=w356:errorcluster, "VElement"=w355:variant)  [unwired: 6 in, 1 out]
          n132 = Variant To Data(error in=w356, type="", Variant=w355) -> (data=w353:string, error out=w352:errorcluster)
          n133 = Scan From String(input string=w363, default 1=Instrument_Types--enum."DAQ" ("Type")) -> (output 1=w362:T6)  [unwired: 3 in, 3 out]
          n134 = case shown="Default" w360 {
            selector: w360 -> [_ w382]
            tunnel: w353 -> [_ w392]
            tunnel: w368 -> [w376 w396]
            tunnel: [w375 w395] -> w367
            tunnel: w352 -> [w372 w393]
            tunnel: w366 -> [_ w391]
            tunnel: [w373 w394] -> w365
            tunnel: w362 -> [w371 w388]
            tunnel: ["" w382] -> w351
            tunnel: [TRUE w379] -> w350
            frame "" {
              n135 = call "Insert Instrument Class by Name.vi"("error in (no error)"=w372, "Type"=w371, "Instrument in"=refnum<class "Instrument.lvclass"> refnum, "Control Experiment in"=w376) -> ("error out"=w373:errorcluster, "Control Experiment out"=w375:refnum<class "Control Experiment.lvclass">)  [unwired: 4 in, 2 out]
            }
            frame Default {
              n136 = call "Find Class by Name.vi"("error in (no error)"=w393, "Name"=w382, "Installed Instruments"=w391) -> ("error out"=w389:errorcluster, "Found?"=w381:bool, "Instrument out"=w390:refnum<class "Instrument.lvclass">)  [unwired: 6 in]
              n137 = call <userlib>:"Write SMO Address.vi"("error in (no error)"=w389, "Address"=w392, "Instrument in"=w390) -> ("error out"=w384:errorcluster, "Instrument out"=w387:refnum<class "Instrument.lvclass">)  [unwired: 7 in]
              n138 = call "Set IsConfigured.vi"("error in (no error)"=w384, "IsConfigured?"=TRUE, "SMO"=w387) -> ("error out"=w383:errorcluster, "SMO out"=w386:refnum<class "Instrument.lvclass">)  [unwired: 7 in]
              n139 = Not(x=w381) -> (.not. x?=w378:bool)
              n140 = call "Insert Instrument Class by Name.vi"("error in (no error)"=w383, "Type"=w388, "Instrument in"=w386, "Control Experiment in"=w396) -> ("error out"=w394:errorcluster, "Found?"=w380:bool, "Control Experiment out"=w395:refnum<class "Control Experiment.lvclass">)  [unwired: 4 in, 1 out]
              n141 = Not(x=w380) -> (.not. x?=w377:bool)
              n142 = Or(x=w377, y=w378) -> (x .or. y?=w379:bool)
            }
          }
        }
        "unresolved" <- w333
        n143 = Bundle By Name(cluster=w343, "C.E."=w341) -> (w344:T7)
        n144 = Merge Errors(w342) -> (w345:errorcluster)
        n145 = call <vilib>:"Add State(s) to Queue__jki_lib_state_machine.vi"("State(s) in (\"\")"=w349) -> ("States Out"=w348:string)  [unwired: 14 in]
      }
    }
  }
  n146 = local read "unresolved"() -> (w1:string[])
  n147 = Unbundle By Name(w9) -> ("C.E."=w7:refnum<class "Control Experiment.lvclass">)
  n148 = Empty Array?(array=w1) -> (empty?=w3:bool)
  n149 = case shown="True" w3 {
    tunnel: w7 -> [_ w407]
    tunnel: [w403 w406] -> w6
    tunnel: w5 -> [w402 w405]
    tunnel: [w402 w404] -> w4
    tunnel: "C.E." -> [w403 _]
    tunnel: w1 -> [w401 _]
    frame False {
      n150 = call <vilib>:"1D String Array to Delimited String.vi"("delimiter"="\n", "string array"=w401) -> ("delimited string"=w399:string)  [unwired: 9 in]
      n151 = Concatenate Strings("Unresolved Instruments:\n" ("string"), w399) -> (w398:string)
      n152 = One Button Dialog(message=w398) -> ()  [unwired: 1 in, 1 out]
    }
    frame True {
      n153 = call "Control Experiment Class to JSON.vi"("error in (no error)"=w405, "Control Experiment in"=w407) -> ("error out"=w404:errorcluster, "Control Experiment out"=w406:refnum<class "Control Experiment.lvclass">)  [unwired: 7 in, 1 out]
    }
  }
  "Control Experiment" <- w6
  "error out" <- w4
